vi "Is_Atomic_Parent.vi"(8 "error in (no error)":errorcluster, 11 "AB_Source in":refnum<class "AB_Source.lvclass">) -> (0 "error out":errorcluster, 1 "autoAdd":bool, 2 "atomicContainer":bool, 3 "AB_Source out":refnum<class "AB_Source.lvclass">)   [LabVIEW 2020, in "AB_Source.lvclass"]
uses:
  <vilib>/AppBuilder/AB_Classes/Source/AB_Source.lvclass
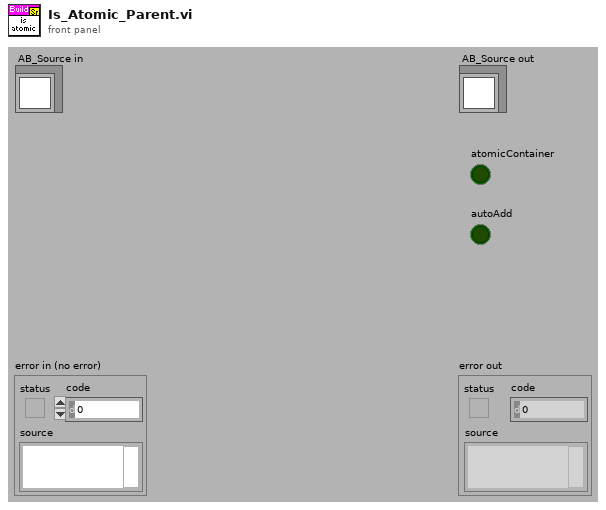
[diagram p1: front panel]
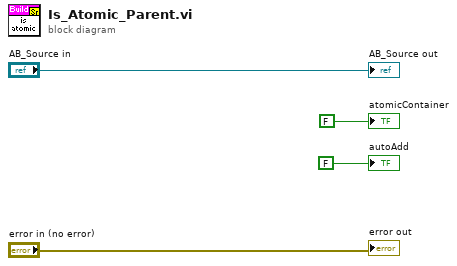
[diagram p0: block diagram]
diagram:
  "error out" <- "error in (no error)"
  "AB_Source out" <- "AB_Source in"
  "atomicContainer" <- FALSE ("atomicContainer?")
  "autoAdd" <- FALSE ("autoAdd")
